vi "ADS1256 Read.vi"(10 "Channel":i8, 11 "DevIndex":i32) -> (2 "function return":i32, 3 "pData":i32[](array[numeric]))   [LabVIEW 2010, in "usb2ads1256.lvlib"]
doc: "int WINAPI ADS1256_Read(int DevIndex,char Channel,int *pData);"
uses:
  usb2ads1256.lvlib
  USB2XXX.dll
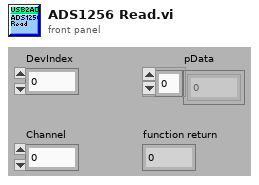
[diagram p1: front panel]
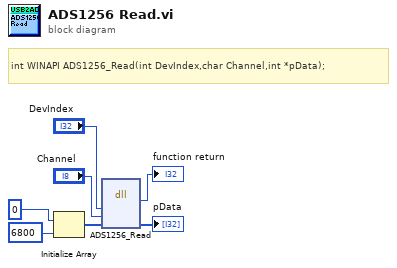
[diagram p0: block diagram]
diagram:
  # "int WINAPI ADS1256_Read(int DevIndex,char Channel,int *pData);"
  n1 = Initialize Array(0 ("element"), 6800 ("dimension size")) -> (w4:i32[])
  n2 = dll-call lib="F:/OtherWork/STM32/USB2XXX_Example/trunk/Labview/PublicFiles/usb2ads1256/USB2XXX.*" fn="ADS1256_Read"("DevIndex"="DevIndex", "Channel"="Channel", "pData"=w4) -> (→"function return":i32, "pData"=→"pData":i32[])  [unwired: 5 in, 2 out]
